vi "publisher.vi"() -> ()   [LabVIEW 2016]
uses:
  <userlib>/ROS for LabVIEW Software/ROS/Code/Console/Servers/ServerSubs/TopicDef.ctl
  <userlib>/ROS for LabVIEW Software/ROS/Code/SubVIs/_ROSDirection.ctl
panel:
  in  "from_rio":cluster{"speed_is":dbl, "steering_is":dbl}
  in  "Publish?":bool
  out "error out":errorcluster
  in  "stop":bool
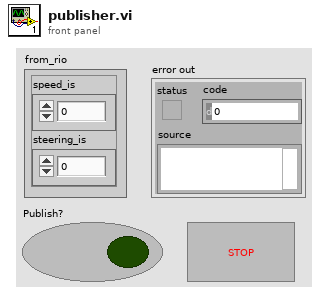
[diagram p1: front panel]
types:
  T1 = typedef "TopicDef.ctl" = cluster{"Topic":string, "Type":string, "Action":T2, "Update (ms)":u16, "queue size":u16}
  T2 = typedef "_ROSDirection.ctl" = enum16{"Node", "Publisher", "Subscriber", "ServiceClient", "ServiceProvider"}
  T3 = typedef "_ROSControl.ctl" = cluster{"topic port":u16, "Node":string, "topic":string, "type":string, "node port":u16, "error ":errorcluster, "Direction":T2, "Update (ms)":u16, "FIFO size":u16}
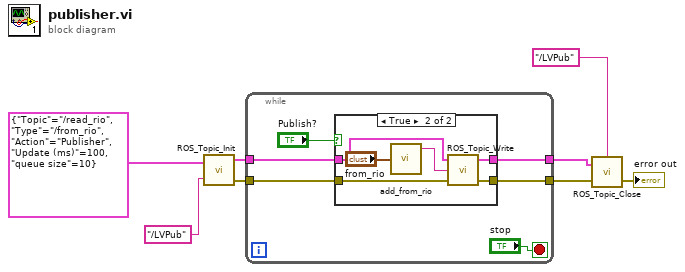
[diagram p0: block diagram]
diagram:
  n1 = call <userlib>:"ROS_Topic_Init.vi"("Definitions"=T1 {"Topic"="/read_rio", "Type"="/from_rio", "Action"=enum."Publisher", "Update (ms)"=100, "queue size"=10}, "node"="/LVPub") -> ("ROS out"=w8:T3, "error out"=w7:errorcluster)  [unwired: 1 in]
  n2 = while {
    tunnel: w8 -> [w14]
    tunnel: w7 -> [w13]
    tunnel: [w11] -> w6
    tunnel: [w10] -> w5
    stop <- "stop" stop-if-true
    n3 = case shown="True" "Publish?" {
      tunnel: w14 -> [w16 w22]
      tunnel: w13 -> [w15 w21]
      tunnel: [w15 w20] -> w11
      tunnel: [w16 w19] -> w10
      frame False {
      }
      frame True {
        n4 = call "add_from_rio.vi"("from_rio"="from_rio") -> ("msg out"=w18:string)  [unwired: 4 in]
        n5 = call <userlib>:"ROS_Topic_Write.vi"("error in (no error)"=w21, "Msg in"=w18, "ROS in"=w22) -> ("error out"=w20:errorcluster, "ROS out"=w19:T3)  [unwired: 1 in]
      }
    }
  }
  n6 = call <userlib>:"ROS_Topic_Close.vi"("error in"=w6, "ROS in"=w5, "node"="/LVPub") -> ("error out"=→"error out":errorcluster)  [unwired: 1 in]
